vi "Purge Dialog.vi"(8 "error in":errorcluster, 11 "Potting Procedure in":refnum<class "Potting Procedure.lvclass">) -> (0 "error out":errorcluster, 2 "Canceled":bool, 3 "Potting Procedure out":refnum<class "Potting Procedure.lvclass">)   [LabVIEW 2011]
uses:
  Procedure Classes/Potting Procedure/Potting Procedure.lvclass
panel:
  in  "OK Button":bool
  in  "Cancel Button":bool
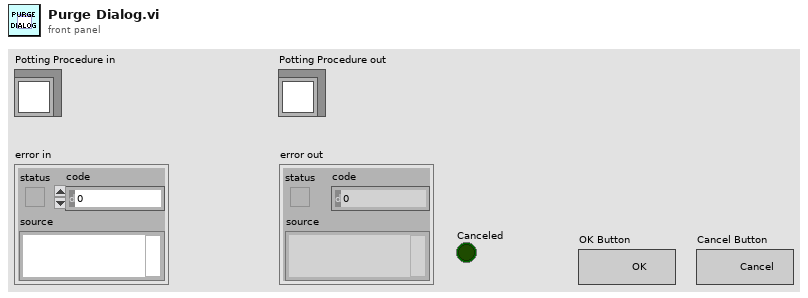
[diagram p1: front panel]
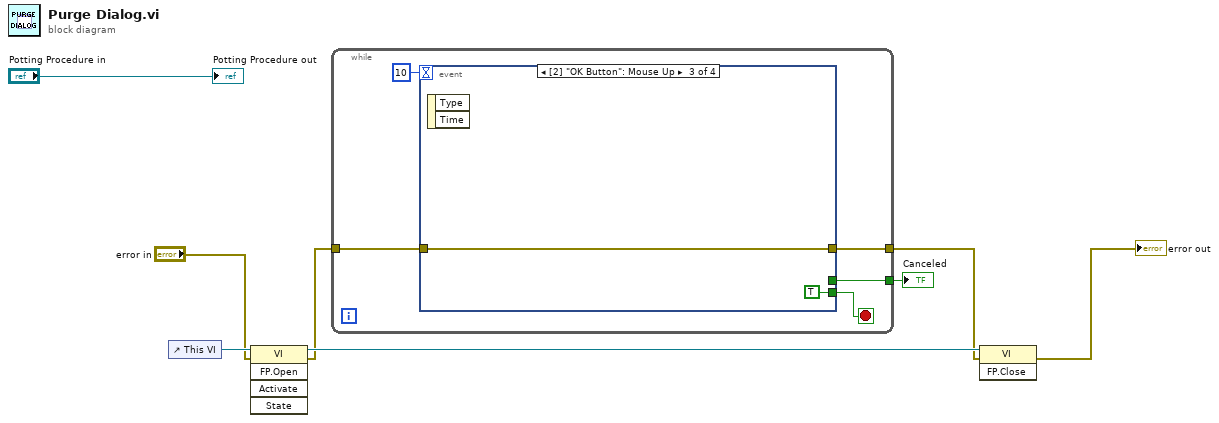
[diagram p0: block diagram]
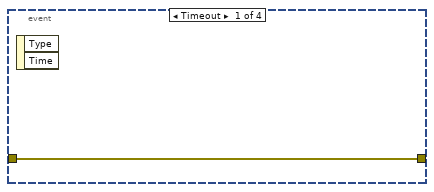
[diagram p2: hidden frame]
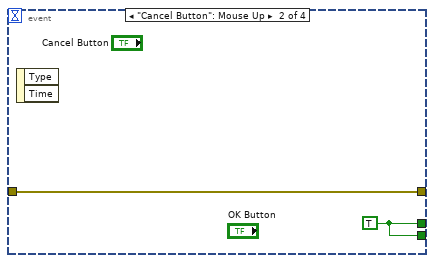
[diagram p3: hidden frame]
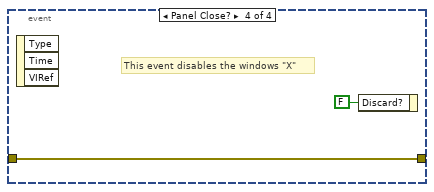
[diagram p4: hidden frame]
diagram:
  n1 = control-ref of="This VI"() -> (w8:refnum<vi>)
  n2 = invoke class="VI" method="FP.Open"(reference=w8, error in="error in") -> (reference out=w7:refnum<vi>, error out=w3:errorcluster)  [unwired: 3 in, 3 out]
  n3 = while {
    tunnel: [w9] -> w4
    tunnel: w3 -> [w10]
    tunnel: [w11] -> w2
    stop <- w12 stop-if-true
    n4 = event shown="[2] \"OK Button\": Mouse Up" {
      selector: _ -> [_ _ _ _]
      dyn-events: _ -> [_ _ _ _]
      timeout: 10 -> [_ _ _ _]
      tunnel: [_ w15 TRUE _] -> w12
      tunnel: [w14 w16 w18 w19] -> w11
      tunnel: w10 -> [w14 w16 w18 w19]
      tunnel: [_ w15 _ _] -> w9
      event Timeout {
        n5 = event-data() -> ()  [unwired: 1 in, 2 out]
      }
      event "Cancel Button": Mouse Up {
        w15 = TRUE
        n6 = event-data() -> ()  [unwired: 1 in, 2 out]
      }
      event "OK Button": Mouse Up {
        n7 = event-data() -> ()  [unwired: 1 in, 2 out]
      }
      event Panel Close? {
        # "This event disables the windows \"X\""
        n8 = event-data() -> ()  [unwired: 1 in, 3 out]
        n9 = event-data("Discard?"=FALSE) -> ()  [unwired: 1 in, 1 out]
      }
    }
  }
  "Canceled" <- w4
  n10 = invoke class="VI" method="FP.Close"(reference=w7, error in=w2) -> (error out=→"error out":errorcluster)  [unwired: 1 in, 2 out]
  "Potting Procedure out" <- "Potting Procedure in"
